vi "Configure System.vi"(0 "VISA resource name":refnum<visa-resource-name>, 1 "DUT Type (0: Amplifier)":i32(ring) items=["Amplifier", "Downconverter", "Upconverter"], 5 "System Fixed LO Frequency (30 GHz)":dbl=30000000000.0 format="%^#_6g", 7 "System Frequency Context (0: RF)":i32(ring) items=["RF", "IF"], 9 "System LO Offset (0: Lower Sideband)":i32(ring) items=["Lower Sideband", "Upper Sideband", "Double Sideband"], 11 "error in (no error)":errorcluster, 12 "Enable System Downconverter (Disabled)":bool) -> (4 "VISA resource name out":refnum<visa-resource-name>, 15 "error out":errorcluster)   [LabVIEW 2014, in "Agilent ESA PSA Series.lvlib"]
doc: "Configures the system options of the Noise Figure personality.\n\n<B>Note:</B> \n\nThis VI is only valid in Noise Figure personality. Use <B>Switch Personality</B> VI to switch to Noise Figure before calling this VI."
uses:
  Agilent ESA PSA Series.lvlib
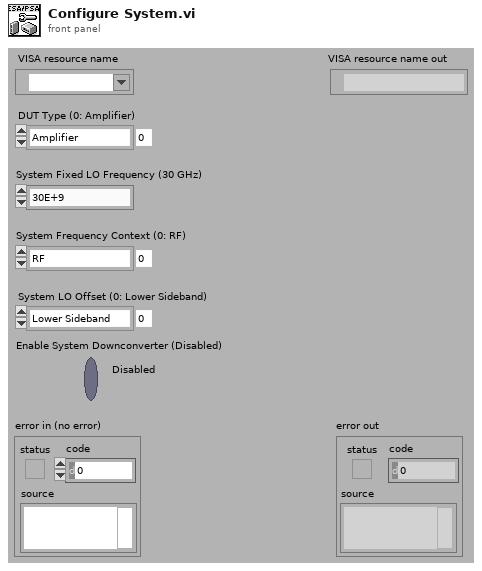
[diagram p1: front panel]
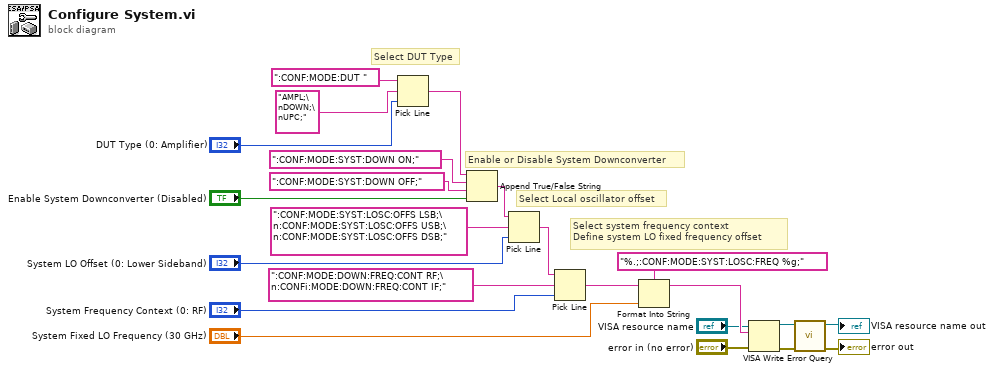
[diagram p0: block diagram]
diagram:
  # "Select system frequency context\nDefine system LO fixed frequency offset"
  # "Select Local oscillator offset"
  # "Enable or Disable System Downconverter"
  # "Select DUT Type"
  n1 = Pick Line(string ("")=":CONF:MODE:DUT ", multi-line string="AMPL;\nDOWN;\nUPC;", line index="DUT Type (0: Amplifier)") -> (output string=w8:string)
  n2 = Append True/False String(1:"Enable System Downconverter (Disabled)", 2:":CONF:MODE:SYST:DOWN OFF;" ("false string"), 3:":CONF:MODE:SYST:DOWN ON;" ("true string"), 4:w8) -> (0:w5:string)
  n3 = Pick Line(string ("")=w5, multi-line string=":CONF:MODE:SYST:LOSC:OFFS LSB;\n:CONF:MODE:SYST:LOSC:OFFS USB;\n:CONF:MODE:SYST:LOSC:OFFS DSB;", line index="System LO Offset (0: Lower Sideband)") -> (output string=w10:string)
  n4 = Pick Line(string ("")=w10, multi-line string=":CONF:MODE:DOWN:FREQ:CONT RF;\n:CONFi:MODE:DOWN:FREQ:CONT IF;", line index="System Frequency Context (0: RF)") -> (output string=w11:string)
  n5 = Format Into String(format string="%.;:CONF:MODE:SYST:LOSC:FREQ %g;", initial string=w11, "System Fixed LO Frequency (30 GHz)") -> (resulting string=w18:string)  [unwired: 1 in, 1 out]
  n6 = VISA Write(VISA resource name="VISA resource name", write buffer=w18, error in (no error)="error in (no error)") -> (VISA resource name out=w21:refnum<visa-resource-name>, error out=w20:errorcluster)  [unwired: 1 out]
  n7 = call "Error Query.vi"("error in (no error)"=w20, "VISA resource name"=w21) -> ("error out"=→"error out":errorcluster, "VISA resource name out"=→"VISA resource name out":refnum<visa-resource-name>)  [unwired: 6 in, 2 out]
